vi "UnusedTest.vi"() -> ()   [LabVIEW 2019, in "TestSuiteTest.lvlib" / "Support.lvlib" / "FakeLibrary.lvlib" / "NestedPrivateLibrary.lvlib"]
uses:
  NestedPrivateLibrary.lvlib
panel:
  out "error out":errorcluster
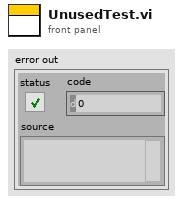
[diagram p1: front panel]
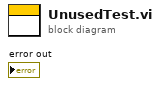
[diagram p0: block diagram]
diagram:
